vi "STAGE+mono+counter_edit23.vi"() -> ()   [LabVIEW 2017]
panel:
  out "Timeout":bool
  out "PROGRESS":u8(slide) max=10 step=10 scale=0.0..1.0
  in  "?":enum32{"Scan Data", "Scans", "RT Data"}(tab)
  out "Spectrum":cluster{dbl[], dbl[]}(graph)
  out "Decay":cluster{dbl[], dbl[]}[](graph)
  in  "Collect Data!":bool
  out "Waveform Graph":waveform(dbl)[](graph)
  out "?":i32(knob) scale=0.0..1000000.0
  out "Photon Counts":dbl
  in  "Wavelength":dbl
  in  "Show Real Time Data":bool
  in  "?":enum32{"DELAY", "COUNTER", "MONO", "PLOT"}(tab)
  in  "Data File Path":path
  out "Final time [ps]":dbl
  out "Current time [ps]":dbl
  out "Initial time [ps]":dbl
  in  "Set this as t0":bool
  in  "Axis":i32=1
  in  "Motor ON":bool
  in  "Motor OFF":bool
  out "Current Position [mm]":dbl
  out "Final Position [mm]":dbl
  in  "Data Points":i32=100
  out "Current Point":i32
  in  "Step Size [um]":i32=10
  in  "Target [mm]":dbl format="%.3f"
  in  "Move":bool
  out "Initial position [mm]":dbl
  in  "GPIB address":string="23"
  in  "Count Mode":u16(ring) items=["A,B for Preset T", "A-B for Preset T", "A+B for Preset T", "A for Preset B"]
  in  "Trigger mode":u16(ring) items=["10 MHz"=0, "Input 2"=2, "Input T"=3]
  in  "Channel A Input":u16(ring)=1 items=["10 MHz", "Input 1"]
  in  "Channel B Input":u16(ring)=2 items=["Input 1"=1, "Input 2"=2]
  in  "Number of Measurements\n to take at one point/ Number of Periods":u16=1 min=1 max=2000 step=1
  in  "Time between measurements\n at one point (s)/Dwell Time":dbl=0.002 min=0.002 max=60.0 step=0.001
  in  "gate mode (CW:0)":i16(slide) scale=0.0..2.0 scale format="%.2f"
  out "Counts":i32
  in  "Integrating time \nin 10^-7 sec":dbl=10000000.0
  in  "Discriminator Level (mV)":dbl min=-300.0 max=300.0 step=0.2
  in  "Discriminator Slope":bool
  in  "Channel":i16 min=0 max=2 step=1
  out "Grating #":dbl
  out "Blaze angle":dbl
  out "Grooves/mm":dbl
  out "Mono port":T1(ring)
  out "Time delay":u32=450000 min=1
  in  "Step size":dbl=10.0 min=0.0
  in  "Scan to":i32=4000
  in  "Scan from":i32=2600
  out "Current wavelength":dbl
  in  "?":bool
  in  "Array":dbl[](array[numeric])
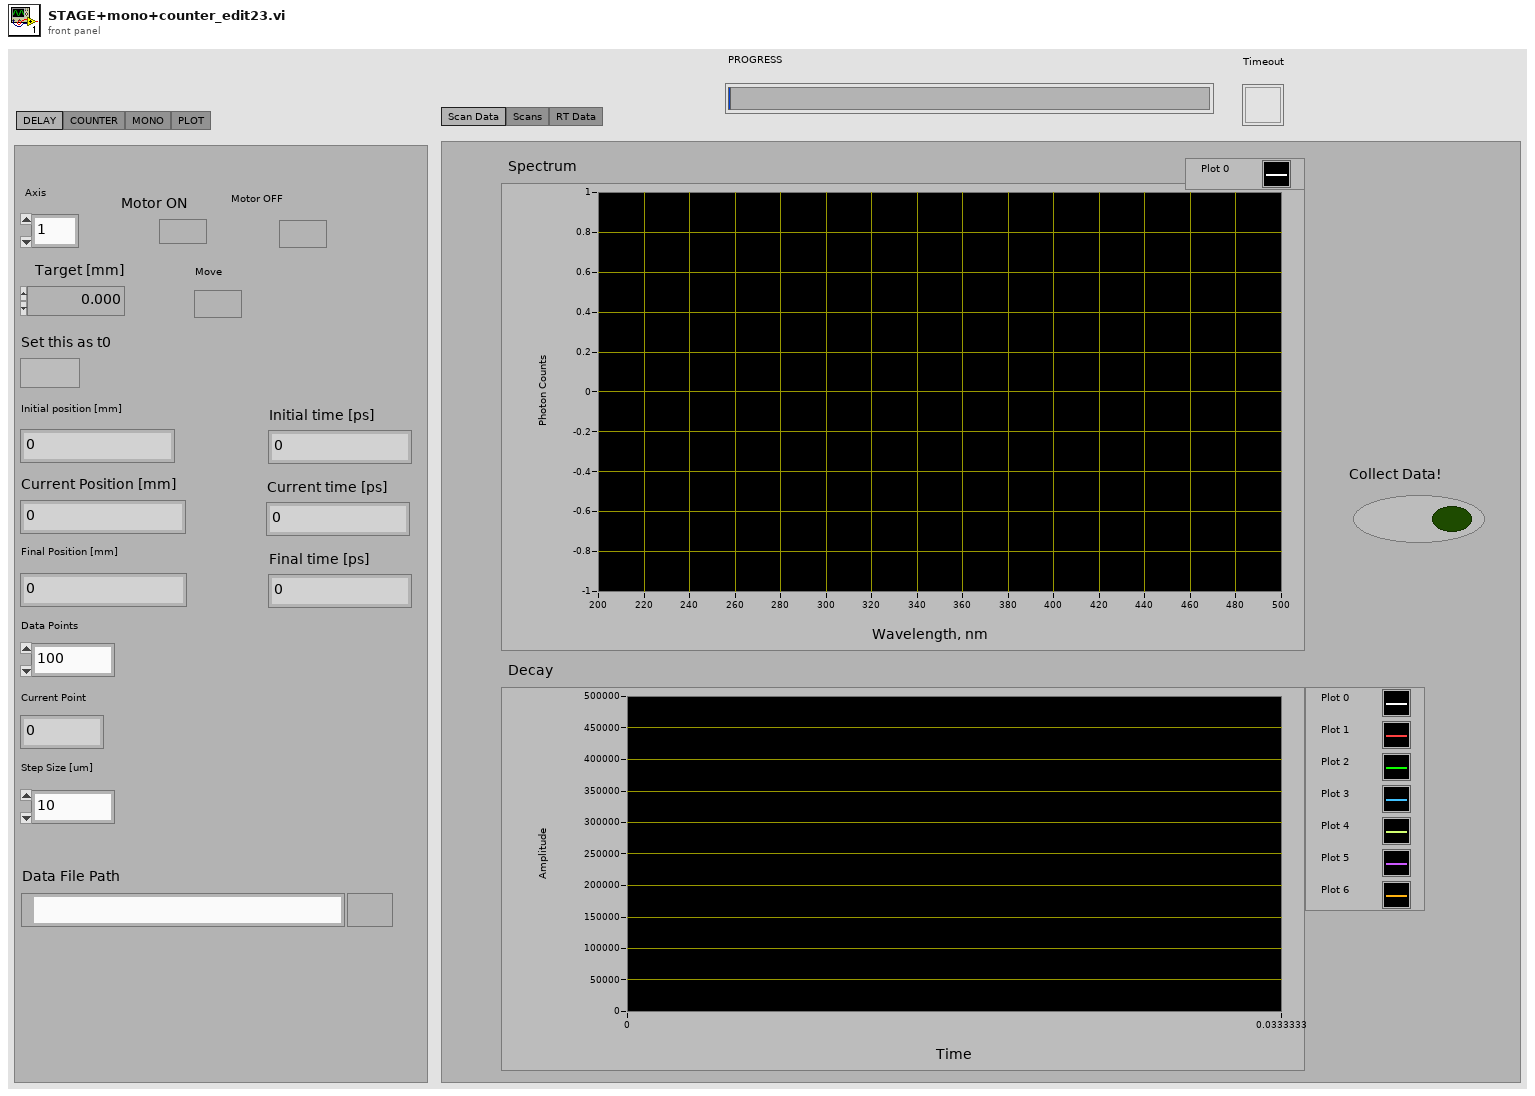
[diagram p1: front panel]
types:
  T1 = enum8{"COM 1", "COM 2", "COM 3", "COM 4", "COM 5", "COM 6", "COM 7", "COM 8", "COM 9"}
  T2 = cluster{"input XON/XOFF":bool, "input HW Handshake":bool, "input alt HW HShk":bool, "output XON/XOFF":bool, "output HW Handshake":bool, "output alt HW HShk":bool, "XOFF byte":u8, "XON byte":u8, "parity error byte":u16}
  T3 = enum16{"no parity", "odd parity", "even parity", "mark parity", "space parity"}
  T4 = enum16{"open", "replace", "create", "open or create", "replace or create", "replace or create with confirmation"}
  T5 = typedef "NI_Matrix.lvlib/RealMatrix.ctl" = dbl[][]
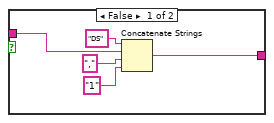
[diagram p3: hidden frame]
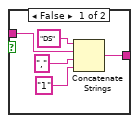
[diagram p5: hidden frame]
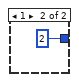
[diagram p9: hidden frame]
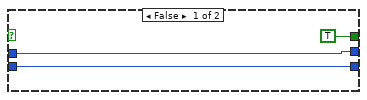
[diagram p10: hidden frame]
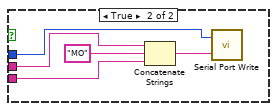
[diagram p11: hidden frame]
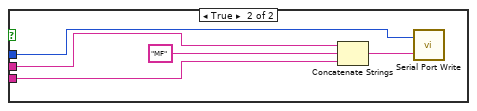
[diagram p12: hidden frame]
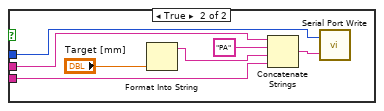
[diagram p13: hidden frame]
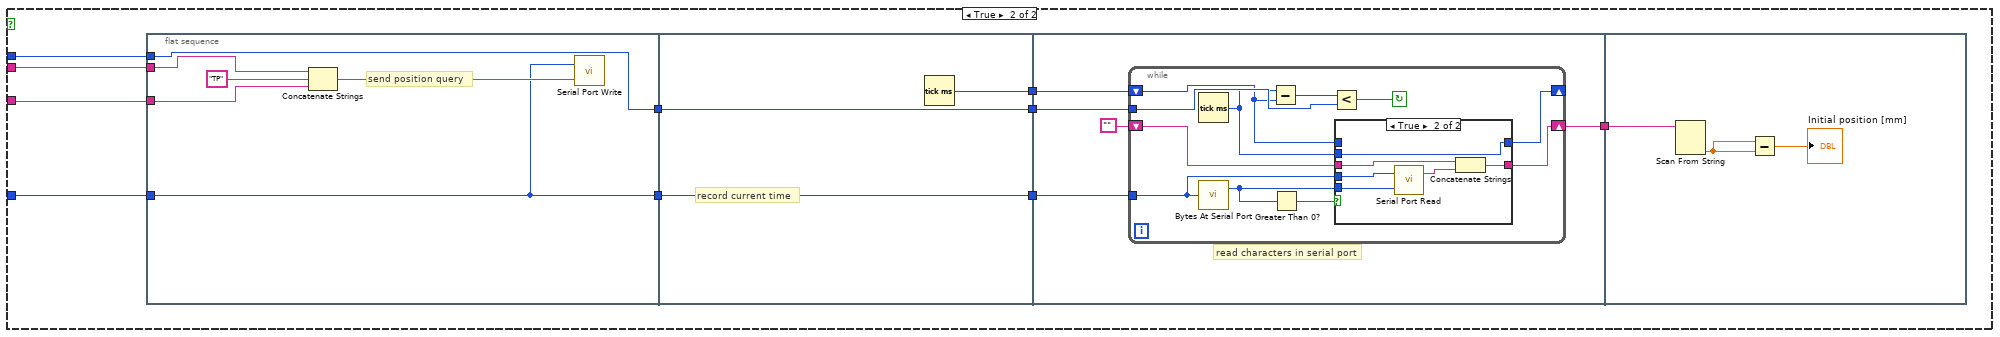
[diagram p14: hidden frame]
diagram:
  (unwired) FALSE
  w28 = u32 19200  # baud rate
  w27 = u16 8  # data bits
  w26 = enum16{"1 bit", "1.5 bits", "2 bits"}."1 bit"  # stop bits
  w30 = T3."no parity"  # parity
  w6 = 4  # 0=COM1 so n=COM(n+1)
  w29 = u16 1024  # buffer size
  n1 = flat-sequence {
    tunnel: [w33] -> w21
    tunnel: [w32] -> w20
    frame #0 {
      n2 = call "CM Com Read ini.vi"() -> ("Mono port"=w32:T1, "time delay1"=w33:u32)  [unwired: 7 in]
    }
  }
  n3 = call "CM Serial Port Setup.vi"("COM port"=w20, "time delay"=w21) -> ("time delay1"=w16:u32, "DK port Out"=w17:T1, "error code"=w19:i32)  [unwired: 7 in]
  n4 = Equal To 0?(x=w19) -> (x = 0?=w18:bool)
  n5 = case shown="True" w18 {
    tunnel: w17 -> [w36 w39]
    tunnel: w16 -> [w35 w38]
    tunnel: [w36 w39] -> w3
    tunnel: [w35 w38] -> w2
    tunnel: [TRUE FALSE] -> w1
    frame False {
    }
    frame True {
      n6 = call "CM Com Write ini.vi"("time delay1"=w39, "Mono port"=w38) -> ()  [unwired: 7 in]
      n7 = local write "Mono port"(w39) -> ()
      n8 = local write "Time delay"(w38) -> ()
    }
  }
  n9 = call <vilib>:"Serial Port Init.vi"("flow control etc."=T2 {"input XON/XOFF"=FALSE, "input HW Handshake"=FALSE, "input alt HW HShk"=FALSE, "output XON/XOFF"=FALSE, "output HW Handshake"=FALSE, "output alt HW HShk"=FALSE, "XOFF byte"=13, "XON byte"=11, "parity error byte"=0}, "parity"=w30, "buffer size"=w29, "stop bits"=w26, "data bits"=w27, "baud rate"=w28, "port number"=w6) -> ("error code"=w25:i32)
  n10 = Concatenate Strings("\r", "\n") -> (w22:string)
  n11 = while {
    tunnel: w2 -> [w42]
    tunnel: w3 -> [w41]
    stop <- TRUE continue-if-true
    n12 = case shown="True" "?" {
      tunnel: w42 -> [_ w45]
      tunnel: w41 -> [_ w44]
      frame False {
      }
      frame True {
        n13 = Two Button Dialog(message="Do you want to change grating?", 1:"No" ("F button name (\"Cancel\")"), 2:"Yes" ("T button name (\"OK\")")) -> (T button?=w46:bool)
        n14 = case shown="True" w46 {
          tunnel: w45 -> [_ w51]
          tunnel: w44 -> [_ w50]
          frame False {
          }
          frame True {
            n15 = Two Button Dialog(message="Disable voltage from PMT", 1:"Do not swich grating" ("F button name (\"Cancel\")"), 2:"Done" ("T button name (\"OK\")")) -> (T button?=w52:bool)
            n16 = case shown="True" w52 {
              tunnel: w51 -> [_ w64]
              tunnel: w50 -> [_ w63]
              frame False {
              }
              frame True {
                n17 = flat-sequence {
                  tunnel: w64 -> [w68]
                  tunnel: [w68] -> w58
                  tunnel: w63 -> [w67]
                  tunnel: [w67] -> w57
                  tunnel: [w65] -> w56
                  tunnel: w58 -> [w73]
                  tunnel: [w73] -> w61
                  tunnel: w57 -> [w74]
                  tunnel: [w74] -> w60
                  tunnel: w56 -> [w72]
                  tunnel: [w72] -> w59
                  tunnel: w61 -> [w78]
                  tunnel: w60 -> [w79]
                  tunnel: [w77] -> w62
                  tunnel: w59 -> [w77]
                  frame #0 {
                    n18 = local read "Grating #"() -> (w66:dbl)
                    n19 = case shown="2, Default" w66 {
                      tunnel: [1 2] -> w65
                      frame 2, Default {
                      }
                      frame 1 {
                      }
                    }
                    n20 = call "Select11x2.vi"("time delay"=w68, "NEW GRT?"=w65, "port number"=w67) -> ()  [unwired: 3 out]
                  }
                  frame #1 {
                    n21 = call "Query11x.vi"("port number"=w74, "QUERY"=u16 2, "time delay"=w73) -> ("STATUS MESSAGE"=w71:u16)  [unwired: 3 out]
                    n22 = local write "Grooves/mm"(w71) -> ()
                  }
                  frame #2 {
                    n23 = Divide(x=w78, y=i16 100 ("device (1)")) -> (x/y=w80:dbl)
                    n24 = call "Query11x.vi"("port number"=w79, "QUERY"=u16 3, "time delay"=w80) -> ("STATUS MESSAGE"=w76:u16)  [unwired: 3 out]
                    n25 = local write "Blaze angle"(w76) -> ()
                  }
                }
                n26 = local write "Grating #"(w62) -> ()
              }
            }
          }
        }
      }
    }
  }
  n27 = while {
    tunnel: w6 -> [w97]
    tunnel: w22 -> [w98]
    tunnel: w25 -> [_]
    tunnel: "Axis" -> [w95]
    stop <- TRUE continue-if-true
    w96 = u32 200  # timeout
    n28 = Format Into String(w95) -> (resulting string=w99:string)  [unwired: 3 in, 1 out]
    n29 = flat-sequence {
      tunnel: w99 -> [w104]
      tunnel: w98 -> [w103]
      tunnel: w97 -> [w105]
      tunnel: w96 -> [w102]
      tunnel: [w104] -> w94
      tunnel: [w103] -> w93
      tunnel: [w105] -> w92
      tunnel: [w102] -> w91
      tunnel: w94 -> [w115]
      tunnel: w93 -> [w114]
      tunnel: w92 -> [w116]
      tunnel: w91 -> [w112]
      tunnel: [w115] -> w90
      tunnel: [w114] -> w89
      tunnel: [w116] -> w88
      tunnel: [w112] -> w87
      tunnel: w90 -> [w125]
      tunnel: w89 -> [w124]
      tunnel: w88 -> [w126]
      tunnel: w87 -> [w122]
      tunnel: [w125] -> w86
      tunnel: [w124] -> w85
      tunnel: [w126] -> w84
      tunnel: [w122] -> w83
      tunnel: w86 -> [w138]
      tunnel: w85 -> [w135]
      tunnel: w84 -> [w137]
      tunnel: w83 -> [w136]
      frame #0 {
        n30 = case shown="False" "Motor ON" {
          tunnel: w105 -> [_ w111]
          tunnel: w104 -> [_ w108]
          tunnel: w103 -> [_ w107]
          frame False {
          }
          frame True {
            n31 = Concatenate Strings(w108, "MO" ("Substring"), w107) -> (w109:string)
            n32 = call <vilib>:"Serial Port Write.vi"("string to write"=w109, "port number"=w111) -> ()  [unwired: 1 out]
          }
        }
      }
      frame #1 {
        n33 = case shown="False" "Motor OFF" {
          tunnel: w116 -> [_ w121]
          tunnel: w115 -> [_ w118]
          tunnel: w114 -> [_ w117]
          frame False {
          }
          frame True {
            n34 = Concatenate Strings(w118, "MF" ("Substring"), w117) -> (w119:string)
            n35 = call <vilib>:"Serial Port Write.vi"("string to write"=w119, "port number"=w121) -> ()  [unwired: 1 out]
          }
        }
      }
      frame #2 {
        n36 = case shown="False" "Move" {
          tunnel: w126 -> [_ w133]
          tunnel: w125 -> [_ w130]
          tunnel: w124 -> [_ w129]
          frame False {
          }
          frame True {
            n37 = Format Into String("Target [mm]") -> (resulting string=w127:string)  [unwired: 3 in, 1 out]
            n38 = Concatenate Strings(w130, "PA" ("Substring"), w127, w129) -> (w131:string)
            n39 = call <vilib>:"Serial Port Write.vi"("string to write"=w131, "port number"=w133) -> ()  [unwired: 1 out]
          }
        }
      }
      frame #3 {
        n40 = case shown="False" "Set this as t0" {
          tunnel: w138 -> [_ w148]
          tunnel: w137 -> [_ w147]
          tunnel: w136 -> [_ w146]
          tunnel: w135 -> [_ w145]
          frame False {
          }
          frame True {
            n41 = flat-sequence {
              tunnel: w148 -> [w152]
              tunnel: w147 -> [w151]
              tunnel: [w151] -> w144
              tunnel: w146 -> [w149]
              tunnel: [w149] -> w143
              tunnel: w145 -> [w150]
              tunnel: w144 -> [w156]
              tunnel: [w156] -> w142
              tunnel: w143 -> [w155]
              tunnel: [w155] -> w141
              tunnel: [w157] -> w140
              tunnel: w142 -> [w162]
              tunnel: w141 -> [w160]
              tunnel: w140 -> [w159]
              tunnel: [w158] -> w139
              tunnel: w139 -> [w184]
              frame #0 {
                # "send position query"
                n42 = Concatenate Strings(w152, "TP" ("Substring"), w150) -> (w153:string)
                n43 = call <vilib>:"Serial Port Write.vi"("string to write"=w153, "port number"=w151) -> ()  [unwired: 1 out]
              }
              frame #1 {
                # "record current time"
                n44 = Tick Count (ms)() -> (millisecond timer value=w157:u32)
              }
              frame #2 {
                # "read characters in serial port"
                n45 = while {
                  shift-left: w159 -> [w163]
                  shift-right: [w164] -> _
                  tunnel: w160 -> [w167]
                  shift-left: "" -> [w170]
                  shift-right: [w169] -> w158
                  tunnel: w162 -> [w171]
                  stop <- w166 continue-if-true
                  n46 = Tick Count (ms)() -> (millisecond timer value=w165:u32)
                  n47 = call <vilib>:"Bytes At Serial Port.vi"("port number"=w171) -> ("byte count"=w172:u32)  [unwired: 1 out]
                  n48 = Subtract(x=w165, y=w163) -> (x-y=w168:u32)
                  n49 = Greater Than 0?(x=w172) -> (x > 0?=w173:bool)
                  n50 = Less?(x=w168, y=w167) -> (x < y?=w166:bool)
                  n51 = case shown="True" w173 {
                    tunnel: w172 -> [_ w181]
                    tunnel: w171 -> [_ w180]
                    tunnel: w170 -> [w175 w178]
                    tunnel: [w175 w177] -> w169
                    tunnel: [w174 w176] -> w164
                    tunnel: w165 -> [_ w176]
                    tunnel: w163 -> [w174 _]
                    frame False {
                    }
                    frame True {
                      n52 = call <vilib>:"Serial Port Read.vi"("requested byte count"=w181, "port number"=w180) -> ("string read"=w179:string)  [unwired: 1 out]
                      n53 = Concatenate Strings(w178, w179) -> (w177:string)
                    }
                  }
                }
              }
              frame #3 {
                n54 = Scan From String(input string=w184) -> (output 1=w182:dbl)  [unwired: 4 in, 3 out]
                n55 = Subtract(x=w182, y=w182) -> (x-y=→"Initial position [mm]":dbl)
              }
            }
          }
        }
      }
    }
    n56 = Wait Until Next ms Multiple(millisecond multiple=u32 50) -> ()  [unwired: 1 out]
  }
  n57 = while {
    tunnel: "GPIB address" -> [w188]
    tunnel: w3 -> [w187]
    tunnel: w2 -> [w186]
    tunnel: w1 -> [w185]
    stop <- TRUE continue-if-true
    n58 = case shown="True" "Show Real Time Data" {
      tunnel: w188 -> [_ w197]
      tunnel: w187 -> [_ w194]
      tunnel: w186 -> [_ w191]
      tunnel: w185 -> [_ w196]
      frame False {
      }
      frame True {
        n59 = flat-sequence {
          tunnel: w197 -> [w226]
          tunnel: "Wavelength" -> [w227]
          tunnel: [w227] -> w208
          tunnel: [w215] -> w207
          tunnel: [w216] -> w206
          tunnel: [w226] -> w205
          tunnel: w191 -> [w216]
          tunnel: w194 -> [w215]
          tunnel: w196 -> [_]
          tunnel: [w214] -> w192
          tunnel: w191 -> [w214]
          tunnel: [w235] -> w204
          tunnel: [w234] -> w203
          tunnel: [w232] -> w202
          tunnel: w208 -> [w230]
          tunnel: w207 -> [w235]
          tunnel: w206 -> [w234]
          tunnel: w205 -> [w232]
          tunnel: [w228] -> w193
          tunnel: w192 -> [w228]
          tunnel: w204 -> [_]
          tunnel: w203 -> [_]
          tunnel: w202 -> [w238]
          tunnel: [w238] -> w201
          tunnel: w194 -> [w237]
          tunnel: w193 -> [w236]
          tunnel: w201 -> [w247]
          tunnel: [w247] -> w200
          tunnel: w200 -> [w297]
          tunnel: [w297] -> w199
          tunnel: w199 -> [w298]
          tunnel: [w298] -> w198
          tunnel: w198 -> [w308]
          frame #0 {
            n60 = call "Query11x.vi"("port number"=w215, "QUERY"=u16 0, "time delay"=w216) -> ("timeout"=w212:bool, "STATUS MESSAGE"=w211:u16)  [unwired: 2 out]
            n61 = call "Query11x.vi"("port number"=w215, "QUERY"=u16 4, "time delay"=w216) -> ("timeout"=w217:bool, "STATUS MESSAGE"=w218:u16)  [unwired: 2 out]
            n62 = call "Query11x.vi"("port number"=w215, "QUERY"=u16 2, "time delay"=w216) -> ("timeout"=w224:bool, "STATUS MESSAGE"=w223:u16)  [unwired: 2 out]
            n63 = call "Query11x.vi"("port number"=w215, "QUERY"=u16 3, "time delay"=w216) -> ("timeout"=w221:bool, "STATUS MESSAGE"=w220:u16)  [unwired: 2 out]
            n64 = local write "Grating #"(w218) -> ()
            n65 = local write "Timeout"(w212) -> ()
            n66 = local write "Timeout"(w224) -> ()
            n67 = local write "Grooves/mm"(w223) -> ()
            n68 = local write "Timeout"(w221) -> ()
            n69 = local write "Blaze angle"(w220) -> ()
            n70 = local write "Timeout"(w217) -> ()
            n71 = Divide(x=w211, y=10 ("Numeric")) -> (x/y=w209:dbl)
            n72 = local write "Current wavelength"(w209) -> ()
          }
          frame #1 {
            n73 = Multiply(x=w230, y=1) -> (x*y=w229:dbl)
            n74 = call "Goto11x.vi"("time delay"=w234, "WAVELENGTH"=w229, "port number"=w235) -> ("timeout"=w233:bool)  [unwired: 2 out]
            n75 = local write "Timeout"(w233) -> ()
          }
          frame #2 {
            # "set counter time in 10^-7 seconds in CW"
            n76 = call "Query11x.vi"("port number"=w237, "QUERY"=0, "time delay"=w236) -> ("timeout"=w242:bool, "STATUS MESSAGE"=w241:u16)  [unwired: 2 out]
            n77 = local write "Timeout"(w242) -> ()
            n78 = Divide(x=w241, y=1) -> (x/y=w240:dbl)
            n79 = local write "Current wavelength"(w240) -> ()
          }
          frame #3 {
            # "Configures discriminator."
            n80 = flat-sequence {
              tunnel: w247 -> [w254]
              tunnel: [w254] -> w253
              tunnel: [w261] -> w252
              tunnel: [w259] -> w251
              tunnel: w246 -> [w260]
              tunnel: w253 -> [w259]
              tunnel: w248 -> [w258]
              tunnel: w252 -> [w280]
              tunnel: [w281] -> w250
              tunnel: w251 -> [w279]
              tunnel: [w279] -> w249
              tunnel: w248 -> [w277]
              tunnel: w250 -> [w293]
              tunnel: w249 -> [w292]
              tunnel: w244 -> [w287]
              tunnel: w248 -> [w286]
              frame #0 {
                # "Flush I/O buffers."
                n81 = for {
                  N: 5 -> [_]
                  tunnel: w254 -> [w256]
                  n82 = GPIB Write(0:w256, 1:"\r") -> ()  [unwired: 3 in, 2 out]
                }
              }
              frame #1 {
                # "Set discriminator slope."
                n83 = case shown="True" w260 {
                  tunnel: [w267 w272] -> w262
                  tunnel: w258 -> [w266 w271]
                  frame False {
                    n84 = Concatenate Strings("DS", w266, ",", "1") -> (w267:string)
                  }
                  frame True {
                    n85 = Concatenate Strings("DS", w271, ",", "0") -> (w272:string)
                  }
                }
                n86 = GPIB Write(0:w259, 1:w262, 2:5) -> (6:w261:errorcluster)  [unwired: 2 in, 1 out]
              }
              frame #2 {
                # "Set discriminator mode to fixed."
                n87 = Concatenate Strings("DM", w277, ",", "0") -> (w276:string)
                n88 = GPIB Write(0:w279, 1:w276, 2:5, 3:w280) -> (6:w281:errorcluster)  [unwired: 1 in, 1 out]
              }
              frame #3 {
                # "Set discriminator level.\nMust be between +300 and -300 mV."
                n89 = Divide(x=w287, y=1000.0) -> (x/y=w295:dbl)
                n90 = Number To Fractional String(number=w295, precision (6)=i16 4) -> (F-format string=w284:string)  [unwired: 2 in]
                n91 = Concatenate Strings("DL", w286, ",", w284) -> (w291:string)
                n92 = GPIB Write(0:w292, 1:w291, 2:5, 3:w293) -> (6:w288:errorcluster)  [unwired: 1 in, 1 out]
                n93 = call <vilib>:"General Error Handler.vi"("type of dialog (OK msg:1)"=1, "error in (no error)"=w288) -> ()  [unwired: 9 in, 5 out]
              }
            }
            n94 = local read "Channel"() -> (w245:i16)
            n95 = local read "Discriminator Slope"() -> (w246:bool)
            n96 = Number To Decimal String(number=w245) -> (decimal integer string=w248:string)  [unwired: 1 in]
            n97 = local read "Discriminator Level (mV)"() -> (w244:dbl)
          }
          frame #4 {
            n98 = call "Start.vi"("GPIB Address"=w297) -> ()  [unwired: 9 in]
          }
          frame #5 {
            # "Wait for Scan to Finish"
            n99 = for {
              N: 1 -> [_]
              tunnel: w298 -> [w300]
              n100 = while {
                tunnel: w300 -> [w301]
                stop <- w303 stop-if-true
                n101 = call "ScanDone.vi"("Wait (ms)"=1000, "GPIB Address"=w301) -> ("Scan Finished?"=w303:bool)
              }
            }
          }
          frame #6 {
            n102 = call "Read Data.vi"("Channel Number"=0, "GPIB Address"=w308, "Number of Datapoints"=1) -> ("Data"=w309:i32[])
            n103 = property class="Knob (strict)"("Scale.Increment"=1000, "Scale.Maximum"=1000000, "Scale.Minimum"=0) -> ()  [unwired: 2 in, 2 out]
            n104 = Index Array(array=w309, index=0) -> (element=→"Photon Counts" →"?":i32)
          }
        }
      }
    }
  }
  n105 = call "Configure.vi"("Dwell Time (s)"="Time between measurements\n at one point (s)/Dwell Time", "Channel T Input"="Trigger mode", "Channel B Input"="Channel B Input", "Channel A Input"="Channel A Input", "Integrating time, 10^-7 sec"="Integrating time \nin 10^-7 sec", "gate mode (CW:0)"="gate mode (CW:0)", "Scan End Mode"=FALSE, "Number of Periods"="Number of Measurements\n to take at one point/ Number of Periods", "Count Mode"="Count Mode", "GPIB Address"="GPIB address") -> ()
  n106 = while {
    tunnel: "Axis" -> [w321]
    tunnel: w6 -> [w320]
    tunnel: "GPIB address" -> [w319]
    tunnel: "Integrating time \nin 10^-7 sec" -> [w318]
    tunnel: w2 -> [w317]
    tunnel: w3 -> [w316]
    tunnel: w1 -> [w315]
    stop <- TRUE continue-if-true
    n107 = case shown="True" "Collect Data!" {
      selector: "Collect Data!" -> [_ w322]
      tunnel: w321 -> [_ w330]
      tunnel: w320 -> [_ w329]
      tunnel: w319 -> [_ w328]
      tunnel: w319 -> [_ w326]
      tunnel: w318 -> [_ w325]
      tunnel: w317 -> [_ w324]
      tunnel: w316 -> [_ w327]
      tunnel: w315 -> [_ w323]
      frame False {
      }
      frame True {
        n108 = flat-sequence {
          tunnel: w330 -> [w350]
          tunnel: w329 -> [w348]
          tunnel: w328 -> [w347]
          tunnel: w327 -> [w346]
          tunnel: w326 -> [w345]
          tunnel: w325 -> [w342]
          tunnel: w324 -> [w335]
          tunnel: w323 -> [w334]
          tunnel: w322 -> [_]
          frame #0 {
            w355 = 1000000000000.0
            w360 = 1000
            w361 = 300000000
            w367 = 1
            n109 = Multiply(x="Step Size [um]", y="Data Points") -> (x*y=w364:i32)
            n110 = Divide(x="Step Size [um]", y=1000.0) -> (x/y=w373:dbl)
            n111 = local read "Initial position [mm]"() -> (w352:dbl)
            n112 = Increment(x="Data Points") -> (x+1=w382:i32)
            n113 = Multiply(x="Scan to", y=w367) -> (x*y=w341:i32)
            n114 = Multiply(x="Scan from", y=w367) -> (x*y=w340:i32)
            n115 = Divide(x=w364, y=1000) -> (x/y=w363:dbl)
            n116 = To Time Stamp(1:w340) -> (0:w370:timestamp)
            n117 = Multiply(x=w341, y=1) -> (x*y=w379:i32)
            n118 = Multiply(x=1, y=w340) -> (x*y=w344:i32)
            n119 = Divide(x=w373, y=1000.0) -> (x/y=w374:dbl)
            n120 = for {
              N: w382 -> [_]
              tunnel: w373 -> [w747]
              tunnel: w352 -> [w745]
              tunnel: [w738] -> w381 mode=indexing
              i -> [w746]
              # "distances"
              n121 = Multiply(x=w747, y=w746) -> (x*y=w744:dbl)
              n122 = Add(x=w745, y=w744) -> (x+y=w743:dbl)
              n123 = Divide(x=w743, y=1000) -> (x/y=w737:dbl)
              n124 = Divide(x=w737, y=300000000) -> (x/y=w740:dbl)
              n125 = Multiply(x=w740, y=1000000000000.0) -> (x*y=w738:dbl)
            }
            n126 = Subtract(x=w379, y=w344) -> (x-y=w385:i32)
            n127 = Divide(x=w352, y=w360) -> (x/y=w358:dbl)
            n128 = Add(x=w352, y=w363) -> (x+y=w354:dbl)
            "Final Position [mm]" <- w354
            n129 = property on="Waveform Graph" class="WFGraph (strict)"("XScale.Increment"="Step size", "XScale.Maximum"=w341, "XScale.Minimum"=w340) -> ()  [unwired: 2 in, 2 out]
            n130 = Divide(x=w385, y="Step size") -> (x/y=w384:dbl)
            n131 = Divide(x=w358, y=w361) -> (x/y=w357:dbl)
            n132 = Divide(x=w374, y=300000000) -> (x/y=w376:dbl)
            n133 = Divide(x=w354, y=w360) -> (x/y=w359:dbl)
            n134 = Bundle By Name("Y"=dbl[] [], "t0"=w370, "dt"="Step size") -> (w369:waveform(dbl))  [unwired: 1 in]
            n135 = Multiply(x=w376, y=1000000000000.0) -> (x*y=w338:dbl)
            n136 = Divide(x=w359, y=w361) -> (x/y=w356:dbl)
            n137 = Multiply(x=w357, y=w355) -> (x*y=w337:dbl)
            "Initial time [ps]" <- w337
            n138 = Build Array(w369) -> (w333:waveform(dbl)[])
            n139 = Round Toward -Infinity(1:w384) -> (0:w343:dbl)
            n140 = Concatenate Strings("\r", "\n") -> (w349:string)
            n141 = Increment(x=w343) -> (x+1=w372:dbl)
            n142 = Multiply(x=w356, y=w355) -> (x*y=w368:dbl)
            "Final time [ps]" <- w368
            n143 = for {
              N: w372 -> [_]
              tunnel: "Step size" -> [w752]
              tunnel: w344 -> [w750]
              tunnel: [w748] -> _ mode=indexing
              i -> [w751]
              # "wavelengths"
              n144 = Multiply(x=w752, y=w751) -> (x*y=w749:dbl)
              n145 = Add(x=w750, y=w749) -> (x+y=w748:dbl)
            }
            n146 = for {
              N: "Data Points" -> [w409]
              tunnel: w352 -> [w450]
              tunnel: "Step Size [um]" -> [w446]
              tunnel: w350 -> [w443]
              tunnel: w349 -> [w440]
              tunnel: w348 -> [w441]
              tunnel: w347 -> [w439]
              tunnel: w346 -> [w437]
              tunnel: w345 -> [w438]
              tunnel: w344 -> [w400]
              tunnel: "Step size" -> [w432]
              tunnel: w343 -> [w431]
              tunnel: w342 -> [w430]
              tunnel: w341 -> [w395]
              tunnel: w340 -> [w394]
              tunnel: "Step size" -> [w396]
              tunnel: w338 -> [w411]
              tunnel: w337 -> [w428]
              shift-right: [w410] -> _
              shift-left: dbl[] [] -> [w406]
              tunnel: w335 -> [w423]
              tunnel: w346 -> [w422]
              tunnel: w334 -> [w421]
              shift-right: [w416] -> _
              shift-left: w333 -> [w417]
              shift-right: [w404] -> _
              shift-left: dbl[][] [] -> [w403]
              shift-right: [w392] -> _
              shift-left: dbl[][] [] -> [w390]
              i -> [w398]
              w420 = dbl[] []
              n147 = stacked-sequence {
                tunnel: w437 -> [w720]
                tunnel: w438 -> [_]
                frame #0 {
                  n148 = call <vilib>:"Close Serial Driver.vi"("port number"=w720) -> ()  [unwired: 1 out]
                  n149 = GPIB Misc(0:"loc 23" ("command string")) -> ()  [unwired: 1 in, 3 out]
                }
              }
              n150 = property on="Waveform Graph" class="WFGraph (strict)"("XScale.Increment"=w396, "XScale.Maximum"=w395, "XScale.Minimum"=w394) -> ()  [unwired: 2 in, 2 out]
              n151 = Number To Decimal String(number=w430) -> (decimal integer string=w435:string)  [unwired: 1 in]
              n152 = Divide(x=w446, y=1000) -> (x/y=w445:dbl)
              n153 = property on="PROGRESS" class="Slide (strict)"("Scale.Increment"=1, "Scale.Maximum"=w409, "Scale.Minimum"=0) -> ()  [unwired: 2 in, 2 out]
              n154 = Multiply(x=w411, y=w398) -> (x*y=w429:dbl)
              n155 = Add(x=1, y=w398) -> (x+y=→"PROGRESS":i32)
              n156 = Concatenate Strings("CP 2,", w435) -> (w433:string)
              n157 = Add(x=w428, y=w429) -> (x+y=w407:dbl)
              n158 = Multiply(x=w445, y=w398) -> (x*y=w449:dbl)
              n159 = Add(x=w450, y=w449) -> (x+y=w448:dbl)
              n160 = Build Array (concatenate)(w406, w407) -> (w408:dbl[])
              n161 = Format Into String(w443) -> (resulting string=w442:string)  [unwired: 3 in, 1 out]
              n162 = GPIB Write(0:w439, 1:w433, 2:i16 5 ("mode (0)")) -> ()  [unwired: 2 in, 2 out]
              n163 = flat-sequence {
                tunnel: w448 -> [w723]
                tunnel: [w723] -> w444
                tunnel: w440 -> [w725]
                tunnel: w442 -> [w724]
                tunnel: w441 -> [w721]
                tunnel: w444 -> [w734]
                tunnel: [w729] -> w393
                frame #0 {
                  n164 = Format Into String(w723) -> (resulting string=w722:string)  [unwired: 3 in, 1 out]
                  n165 = Wait (ms)(milliseconds to wait=u32 100) -> ()  [unwired: 1 out]
                  n166 = Concatenate Strings(w724, "PA" ("Substring"), w722, w725) -> (w727:string)
                  n167 = call <vilib>:"Serial Port Write.vi"("string to write"=w727, "port number"=w721) -> ()  [unwired: 1 out]
                }
                frame #1 {
                  n168 = Divide(x=w734, y=1000) -> (x/y=w732:dbl)
                  n169 = Wait (ms)(milliseconds to wait=u32 1000) -> ()  [unwired: 1 out]
                  n170 = Divide(x=w732, y=300000000) -> (x/y=w731:dbl)
                  n171 = Multiply(x=w731, y=1000000000000.0) -> (x*y=w729:dbl)
                  "Current time [ps]" <- w729
                  "Current Position [mm]" <- w734
                }
              }
              n172 = Add(x=w398, y=1) -> (x+y=w397:i32)
              n173 = flat-sequence {
                tunnel: w439 -> [w476]
                tunnel: w400 -> [w475]
                tunnel: w432 -> [w474]
                tunnel: w431 -> [w473]
                tunnel: w395 -> [w472]
                tunnel: w394 -> [w471]
                tunnel: w420 -> [w470]
                tunnel: w420 -> [w469]
                tunnel: w396 -> [w468]
                tunnel: w423 -> [w467]
                tunnel: w422 -> [w466]
                tunnel: w421 -> [w465]
                tunnel: [w463] -> w419
                tunnel: [w464] -> _
                tunnel: [w463] -> w418
                tunnel: w397 -> [w462]
                tunnel: w393 -> [w461]
                tunnel: [w460] -> w391
                tunnel: w390 -> [w459]
                tunnel: w419 -> [w698]
                tunnel: [w701] -> w405
                tunnel: [w700] -> w402
                tunnel: [w699] -> w392
                tunnel: w391 -> [w699]
                frame #0 {
                  # "step size"
                  n174 = while {
                    tunnel: w476 -> [w518]
                    tunnel: w475 -> [w539]
                    tunnel: w474 -> [w511]
                    tunnel: w473 -> [w538]
                    tunnel: w472 -> [w514]
                    tunnel: w471 -> [w513]
                    tunnel: w468 -> [w515]
                    shift-right: [w535] -> w463
                    shift-left: w469 -> [w534]
                    shift-right: [w530] -> w464
                    shift-left: w470 -> [w537]
                    tunnel: w467 -> [w477]
                    tunnel: w466 -> [w478]
                    tunnel: w465 -> [w520]
                    tunnel: w462 -> [w499]
                    tunnel: w461 -> [w487]
                    shift-right: [w480] -> w460
                    shift-left: w459 -> [w479]
                    i -> [w507]
                    stop <- w509 stop-if-true
                    n175 = property on="Spectrum" class="XYGraph (strict)"("XScale.Increment"=w515, "XScale.Maximum"=w514, "XScale.Minimum"=w513) -> ()  [unwired: 2 in, 2 out]
                    n176 = Multiply(x=1, y=w511) -> (x*y=w510:dbl)
                    n177 = Multiply(x=w507, y=w510) -> (x*y=w540:dbl)
                    n178 = Greater Or Equal?(x=w507, y=w538) -> (x >= y?=w509:bool)
                    n179 = Add(x=w540, y=w539) -> (x+y=w519:dbl)
                    n180 = Add(x=w507, y=1) -> (x+y=w500:i32)
                    n181 = Build Array (concatenate)(w537, w519) -> (w536:dbl[])
                    n182 = flat-sequence {
                      tunnel: w518 -> [w560]
                      tunnel: w519 -> [w561]
                      tunnel: [w561] -> w524
                      tunnel: [w542] -> w523
                      tunnel: [w541] -> w522
                      tunnel: [w560] -> w521
                      tunnel: w477 -> [w541]
                      tunnel: w478 -> [w542]
                      tunnel: w520 -> [_]
                      tunnel: [w559] -> w501
                      tunnel: w500 -> [w559]
                      tunnel: [w558] -> w488
                      tunnel: w487 -> [w558]
                      tunnel: w479 -> [w557]
                      tunnel: [w557] -> w486
                      tunnel: [w571] -> w529
                      tunnel: [w570] -> w528
                      tunnel: [w568] -> w527
                      tunnel: w524 -> [w564]
                      tunnel: w523 -> [w571]
                      tunnel: w522 -> [w570]
                      tunnel: w521 -> [w568]
                      tunnel: [w565] -> w502
                      tunnel: w501 -> [w565]
                      tunnel: [w564] -> w494
                      tunnel: [w563] -> w489
                      tunnel: w488 -> [w563]
                      tunnel: w486 -> [w562]
                      tunnel: [w562] -> w485
                      tunnel: w529 -> [_]
                      tunnel: w528 -> [_]
                      tunnel: w527 -> [w578]
                      tunnel: [w578] -> w517
                      tunnel: [w577] -> w503
                      tunnel: w502 -> [w577]
                      tunnel: [w576] -> w495
                      tunnel: w494 -> [w576]
                      tunnel: [w575] -> w490
                      tunnel: w489 -> [w575]
                      tunnel: w485 -> [w574]
                      tunnel: [w574] -> w484
                      tunnel: w478 -> [w573]
                      tunnel: w477 -> [w572]
                      tunnel: w517 -> [w588]
                      tunnel: [w588] -> w516
                      tunnel: [w587] -> w504
                      tunnel: w503 -> [w587]
                      tunnel: [w586] -> w496
                      tunnel: w495 -> [w586]
                      tunnel: [w585] -> w491
                      tunnel: w490 -> [w585]
                      tunnel: w484 -> [w584]
                      tunnel: [w584] -> w483
                      tunnel: w516 -> [w645]
                      tunnel: [w645] -> w526
                      tunnel: [w644] -> w505
                      tunnel: w504 -> [w644]
                      tunnel: [w643] -> w497
                      tunnel: w496 -> [w643]
                      tunnel: [w642] -> w492
                      tunnel: w491 -> [w642]
                      tunnel: w483 -> [w641]
                      tunnel: [w641] -> w482
                      tunnel: w526 -> [w650]
                      tunnel: [w650] -> w525
                      tunnel: [w649] -> w506
                      tunnel: w505 -> [w649]
                      tunnel: [w648] -> w498
                      tunnel: w497 -> [w648]
                      tunnel: [w647] -> w493
                      tunnel: w492 -> [w647]
                      tunnel: w482 -> [w646]
                      tunnel: [w646] -> w481
                      tunnel: [w661] -> w532
                      tunnel: w525 -> [w693]
                      tunnel: w506 -> [w659]
                      tunnel: w499 -> [w662]
                      tunnel: w498 -> [w663]
                      tunnel: w493 -> [w665]
                      tunnel: w481 -> [w660]
                      tunnel: [w658] -> w480
                      frame #0 {
                        n183 = call "Query11x.vi"("port number"=w542, "QUERY"=u16 4, "time delay"=w541) -> ("timeout"=w544:bool, "STATUS MESSAGE"=→"Grating #":u16)  [unwired: 2 out]
                        n184 = call "Query11x.vi"("port number"=w542, "QUERY"=u16 3, "time delay"=w541) -> ("timeout"=w547:bool, "STATUS MESSAGE"=→"Blaze angle":u16)  [unwired: 2 out]
                        n185 = call "Query11x.vi"("port number"=w542, "QUERY"=u16 0, "time delay"=w541) -> ("timeout"=w555:bool, "STATUS MESSAGE"=w554:u16)  [unwired: 2 out]
                        n186 = call "Query11x.vi"("port number"=w542, "QUERY"=u16 2, "time delay"=w541) -> ("timeout"=w550:bool, "STATUS MESSAGE"=→"Grooves/mm":u16)  [unwired: 2 out]
                        n187 = local write "Timeout"(w555) -> ()
                        n188 = Divide(x=w554, y=1 ("Numeric")) -> (x/y=→"Current wavelength":dbl)
                        n189 = local write "Timeout"(w544) -> ()
                        n190 = local write "Timeout"(w547) -> ()
                        n191 = local write "Timeout"(w550) -> ()
                      }
                      frame #1 {
                        n192 = Multiply(x=w564, y=1) -> (x*y=w566:dbl)
                        n193 = call "Goto11x.vi"("time delay"=w570, "WAVELENGTH"=w566, "port number"=w571) -> ("timeout"=w569:bool)  [unwired: 2 out]
                        n194 = local write "Timeout"(w569) -> ()
                      }
                      frame #2 {
                        # "set counter time in 10^-7 seconds in CW"
                        n195 = call "Query11x.vi"("port number"=w573, "QUERY"=0, "time delay"=w572) -> ("timeout"=w582:bool, "STATUS MESSAGE"=w581:u16)  [unwired: 2 out]
                        n196 = local write "Timeout"(w582) -> ()
                        n197 = Divide(x=w581, y=1) -> (x/y=w580:dbl)
                        n198 = local write "Current wavelength"(w580) -> ()
                      }
                      frame #3 {
                        # "Configures discriminator."
                        n199 = flat-sequence {
                          tunnel: w588 -> [w598]
                          tunnel: [w598] -> w597
                          tunnel: [w605] -> w596
                          tunnel: [w603] -> w595
                          tunnel: "Discriminator Slope" -> [w604]
                          tunnel: w597 -> [w603]
                          tunnel: w589 -> [w602]
                          tunnel: w596 -> [w624]
                          tunnel: [w625] -> w594
                          tunnel: w595 -> [w623]
                          tunnel: [w623] -> w593
                          tunnel: w589 -> [w621]
                          tunnel: w594 -> [w637]
                          tunnel: w593 -> [w636]
                          tunnel: "Discriminator Level (mV)" -> [w631]
                          tunnel: w589 -> [w630]
                          frame #0 {
                            # "Flush I/O buffers."
                            n200 = for {
                              N: 5 -> [_]
                              tunnel: w598 -> [w600]
                              n201 = GPIB Write(0:w600, 1:"\r") -> ()  [unwired: 3 in, 2 out]
                            }
                          }
                          frame #1 {
                            # "Set discriminator slope."
                            n202 = case shown="True" w604 {
                              tunnel: [w611 w616] -> w606
                              tunnel: w602 -> [w610 w615]
                              frame False {
                                n203 = Concatenate Strings("DS", w610, ",", "1") -> (w611:string)
                              }
                              frame True {
                                n204 = Concatenate Strings("DS", w615, ",", "0") -> (w616:string)
                              }
                            }
                            n205 = GPIB Write(0:w603, 1:w606, 2:5) -> (6:w605:errorcluster)  [unwired: 2 in, 1 out]
                          }
                          frame #2 {
                            # "Set discriminator mode to fixed."
                            n206 = Concatenate Strings("DM", w621, ",", "0") -> (w620:string)
                            n207 = GPIB Write(0:w623, 1:w620, 2:5, 3:w624) -> (6:w625:errorcluster)  [unwired: 1 in, 1 out]
                          }
                          frame #3 {
                            # "Set discriminator level.\nMust be between +300 and -300 mV."
                            n208 = Divide(x=w631, y=1000.0) -> (x/y=w639:dbl)
                            n209 = Number To Fractional String(number=w639, precision (6)=i16 4) -> (F-format string=w628:string)  [unwired: 2 in]
                            n210 = Concatenate Strings("DL", w630, ",", w628) -> (w635:string)
                            n211 = GPIB Write(0:w636, 1:w635, 2:5, 3:w637) -> (6:w632:errorcluster)  [unwired: 1 in, 1 out]
                            n212 = call <vilib>:"General Error Handler.vi"("type of dialog (OK msg:1)"=1, "error in (no error)"=w632) -> ()  [unwired: 9 in, 5 out]
                          }
                        }
                        n213 = Number To Decimal String(number="Channel") -> (decimal integer string=w589:string)  [unwired: 1 in]
                      }
                      frame #4 {
                        n214 = call "Start.vi"("GPIB Address"=w645) -> ()  [unwired: 9 in]
                      }
                      frame #5 {
                        # "Wait for Scan to Finish"
                        n215 = for {
                          N: 1 -> [_]
                          tunnel: w650 -> [w652]
                          n216 = while {
                            tunnel: w652 -> [w653]
                            stop <- w655 stop-if-true
                            n217 = call "ScanDone.vi"("Wait (ms)"=1000, "GPIB Address"=w653) -> ("Scan Finished?"=w655:bool)
                          }
                        }
                      }
                      frame #6 {
                        w664 = 0
                        w672 = "\r\n"
                        n218 = call "Read Data.vi"("Channel Number"=0, "GPIB Address"=w693, "Number of Datapoints"=1) -> ("Data"=w694:i32[])
                        n219 = Index Array(array=w694, index=0) -> (element=w661:i32)
                        "Counts" <- w661
                        n220 = local read "Integrating time \nin 10^-7 sec"() -> (w670:dbl)
                        n221 = Replace Array Subset(array=w660, new element #1=w661, index (row) #1=w659, index (col) #1=w662, new element #2=w663, index (row) #2=w659, index (col) #2=w664, new element #3=w665, index (row) #3=w664, index (col) #3=w662) -> (w658:T5)
                        n222 = Array To Spreadsheet String(delimiter (Tab)=",", array=w658, 3:"%f" ("format string")) -> (spreadsheet string=w671:string)
                        n223 = local read "Blaze angle"() -> (w688:dbl)
                        n224 = local read "Grating #"() -> (w687:dbl)
                        n225 = Multiply(x=w670, y=1e-07) -> (x*y=w669:dbl)
                        n226 = Get Date/Time In Seconds() -> (seconds since 1Jan1904=w682:timestamp)
                        n227 = Format Date/Time String(time format string (%c)="%Y-%b-%d %H:%M:%S", seconds (now)=w682) -> (date/time string=w683:string)  [unwired: 1 in]
                        n228 = Number To Decimal String(number=w669) -> (decimal integer string=w684:string)  [unwired: 1 in]
                        n229 = Number To Decimal String(number=w687) -> (decimal integer string=w685:string)  [unwired: 1 in]
                        n230 = Number To Decimal String(number=w688) -> (decimal integer string=w673:string)  [unwired: 1 in]
                        n231 = call <vilib>:"Space Constant.vi"() -> ("String"=w686:string)
                        n232 = Open/Create/Replace File(file path (use dialog)="Data File Path", operation (0:open)=T4."replace or create") -> (refnum out=w692:refnum<file>)  [unwired: 4 in, 2 out]
                        n233 = Concatenate Strings(w672, "Data was taken on ", w683, w672, "Integration Time is ", w684, w686, "s", w672, "Monochromator gratng # ", w685, "; ", "blazed for ", w673, w686, "nm", w672, w672, w672, w671) -> (w667:string)
                        n234 = Write to Text File(file (use dialog)=w692, text=w667) -> (refnum out=w657:refnum<file>)  [unwired: 2 in, 2 out]
                        n235 = Flush File(refnum=w657) -> (refnum out=w656:refnum<file>)  [unwired: 1 in, 1 out]
                        n236 = Close File(refnum=w656) -> ()  [unwired: 1 in, 2 out]
                      }
                    }
                    n237 = Build Array (concatenate)(w534, w532) -> (w533:dbl[])
                    n238 = Bundle(w536, w533) -> (w531:cluster{dbl[], dbl[]})  [unwired: 1 in]
                    "Spectrum" <- w531
                    n239 = Unbundle(w531) -> (w530:dbl[], w535:dbl[])
                  }
                }
                frame #1 {
                  n240 = Array Size(array="Array") -> (size(s)=w700:i32)
                  n241 = flat-sequence {
                    tunnel: w698 -> [w707]
                    tunnel: "Array" -> [w706]
                    tunnel: w700 -> [w705]
                    tunnel: [w703] -> w701
                    frame #0 {
                      n242 = for {
                        N: w705 -> [_]
                        tunnel: w706 -> [w718]
                        tunnel: w707 -> [w713]
                        shift-right: [w708] -> w703
                        shift-left: dbl[] [] -> [w709]
                        i -> [w711]
                        n243 = local read "Scan from"() -> (w716:i32)
                        n244 = Index Array(array=w718, index=w711) -> (element=w717:dbl)
                        n245 = local read "Step size"() -> (w714:dbl)
                        n246 = Subtract(x=w717, y=w716) -> (x-y=w715:dbl)
                        n247 = Divide(x=w715, y=w714) -> (x/y=w712:dbl)
                        n248 = Index Array(array=w713, index=w712) -> (element=w710:dbl)
                        n249 = Insert Into Array(array=w709, index=w711, new element=w710) -> (w708:dbl[])
                      }
                    }
                  }
                }
              }
              n250 = local read "Scan from"() -> (w414:i32)
              n251 = local read "Step size"() -> (w412:dbl)
              n252 = To Time Stamp(1:w414) -> (0:w413:timestamp)
              n253 = Bundle By Name("Y"=w418, "t0"=w413, "dt"=w412) -> (w415:waveform(dbl))  [unwired: 1 in]
              n254 = Build Array (concatenate)(w417, w415) -> (w416:waveform(dbl)[])
              "Waveform Graph" <- w416
              n255 = for {
                N: w402 -> [_]
                tunnel: [w458] -> w410
                tunnel: w408 -> [w457]
                tunnel: w405 -> [w455]
                tunnel: [w454] -> w404
                tunnel: w403 -> [w456]
                tunnel: [w451] -> w401 mode=indexing
                i -> [w453]
                n256 = Build Array (concatenate)(w456, w455) -> (w454:dbl[][])
                n257 = Index Array(array=w455, index=w453) -> ()  [unwired: 1 out]
                n258 = Index Array(array=w454, index (col)=w453) -> (element=w452:dbl[])  [unwired: 1 in]
                n259 = Bundle(w457, w452) -> (w451:cluster{dbl[], dbl[]})  [unwired: 1 in]
                n260 = Unbundle(w451) -> (w458:dbl[])  [unwired: 1 out]
              }
              "Decay" <- w401
              "Current Point" <- w398
            }
            n261 = property on="Decay" class="XYGraph (strict)"("XScale.Increment"=w338, "XScale.Maximum"=w368, "XScale.Minimum"=w337) -> ()  [unwired: 2 in, 2 out]
            n262 = Build Array (concatenate)(0, w381) -> ()  [unwired: 1 out]
          }
        }
      }
    }
  }
  "Mono port" <- w20
  "Time delay" <- w21
